vi "RF_Synth_send_command.vi"(1 "Value":dbl=3.0, 3 "COM address":string="0:19") -> ()   [LabVIEW 2013]
panel:
  in  "Parameter":T1(ring)
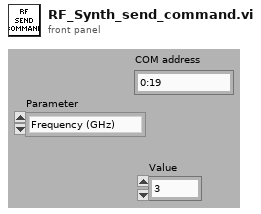
[diagram p1: front panel]
types:
  T1 = enum16{"Frequency (GHz)", "Power (dBm)", "Phase (deg)", "Output on?", "Trigger mode", "Set channel", "Init"}
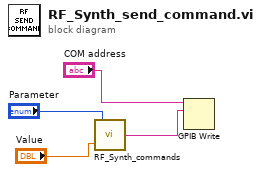
[diagram p0: block diagram]
diagram:
  n1 = call "RF_Synth_commands.vi"("Value"="Value", "Parameter"="Parameter") -> ("Command"=w3:string)
  n2 = GPIB Write(0:"COM address", 1:w3) -> ()  [unwired: 1 in, 4 out]
